vi "addToNewColumn.vi"(9 "disabled index (col)":i32=2, 10 "new file path (Not A Path if cancelled)":path, 11 "Array":dbl[][](array[numeric])) -> ()   [LabVIEW 2012]
uses:
  <vilib>/Utility/file.llb/Read From Spreadsheet File (DBL).vi
  <vilib>/Utility/file.llb/Write To Spreadsheet File (DBL).vi
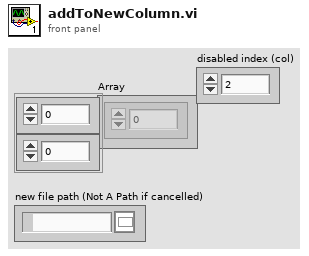
[diagram p1: front panel]
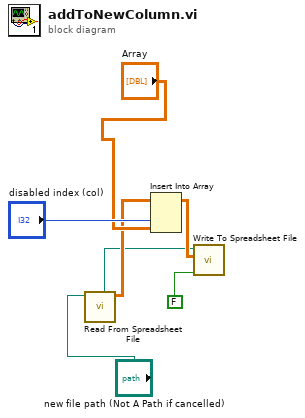
[diagram p0: block diagram]
diagram:
  n1 = call-poly <vilib>:"Read From Spreadsheet File.vi"("file path (dialog if empty)"="new file path (Not A Path if cancelled)") -> ("all rows"=w4:dbl[][], "new file path (Not A Path if cancelled)"=w3:path)  [unwired: 6 in, 3 out]
  n2 = Insert Into Array(array=w4, index (col)="disabled index (col)", new element="Array") -> (w7:dbl[][])  [unwired: 1 in]
  n3 = call-poly <vilib>:"Write To Spreadsheet File.vi"("append to file? (new file:F)"=FALSE, "2D data"=w7, "file path (dialog if empty)"=w3) -> ()  [unwired: 5 in, 1 out]
